vi "Convert String to Hex String.vi"(11 "String":string) -> (3 "Hex String":string)   [LabVIEW 2020, in "MacroAssert.lvlib"]
doc: "Converts <B>String</B> to a hex-coded string."
uses:
  MacroAssert.lvlib
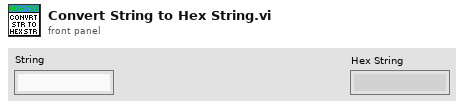
[diagram p1: front panel]
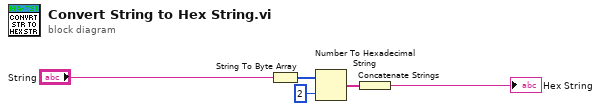
[diagram p0: block diagram]
diagram:
  n1 = String To Byte Array(string="String") -> (unsigned byte array=w5:u8[])
  n2 = Number To Hexadecimal String(1:i16 2 ("width (-)"), 2:w5) -> (0:w4:string[])
  n3 = Concatenate Strings(w4) -> (→"Hex String":string)
